vi "To String.vi"(8 "error in (no error)":errorcluster, 11 "JSON String in":refnum<class "JSON String.lvclass">) -> (0 "error out":errorcluster, 3 "String":string)   [LabVIEW 2015, in "LVJSON.lvlib" / "JSON String.lvclass"]
uses:
  JSON String.lvclass
  JSON String.lvclass/JSON String.ctl
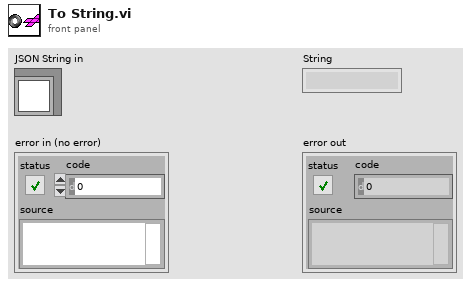
[diagram p1: front panel]
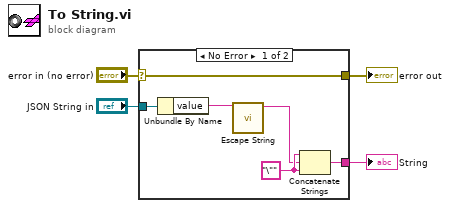
[diagram p0: block diagram]
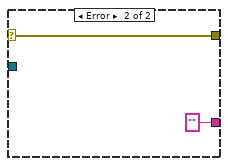
[diagram p2: hidden frame]
diagram:
  n1 = case shown="No Error" "error in (no error)" {
    selector: "error in (no error)" -> [w7 w11]
    tunnel: "JSON String in" -> [w10 _]
    tunnel: [w8 ""] -> w3
    tunnel: [w7 w11] -> w2
    frame No Error {
      w9 = "\"" ("string")
      n2 = Unbundle By Name(w10) -> ("value"=w6:string)
      n3 = call "Escape String.vi"("value"=w6) -> ("escaped string"=w5:string)  [unwired: 10 in]
      n4 = Concatenate Strings(w9, w5, w9) -> (w8:string)
    }
    frame Error {
    }
  }
  "String" <- w3
  "error out" <- w2
